vi "Set AQS.vi"(0 "NMR in":refnum<class "NMR.lvclass">, 5 "Number Samples":u16=5000 step=1, 7 "Units":u8(ring) items=["us", "ms"], 9 "Time Between Points":dbl min=0.0 step=1.0, 11 "error in (no error)":errorcluster) -> (4 "NMR out":refnum<class "NMR.lvclass">, 6 "Real Time":ext, 10 "String as ASCII":string, 15 "error out":errorcluster)   [LabVIEW 2011, in "NMR.lvclass"]
uses:
  NMR.lvclass
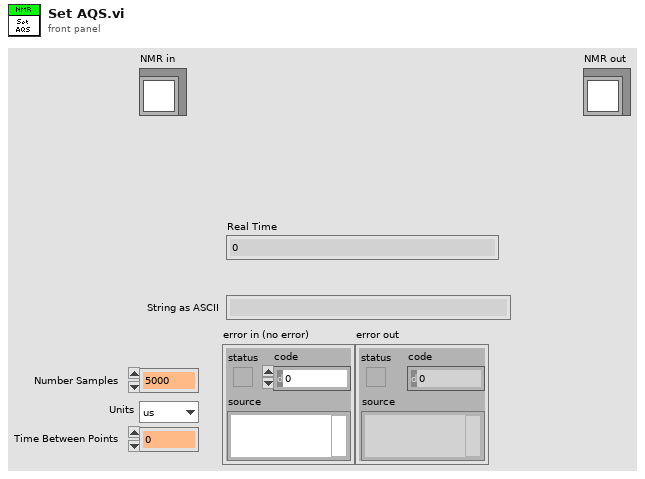
[diagram p1: front panel]
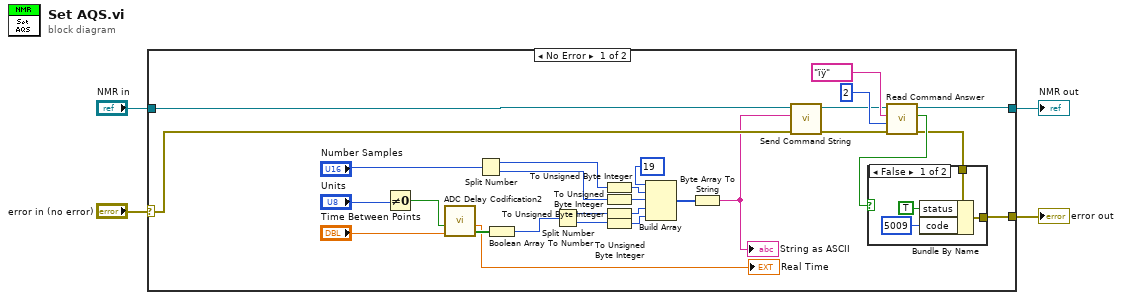
[diagram p0: block diagram]
diagram:
  n1 = case shown="No Error" "error in (no error)" {
    selector: "error in (no error)" -> [w31 w39]
    tunnel: [w5 w39] -> w3
    tunnel: [w7 w38] -> w1
    tunnel: "NMR in" -> [w32 w38]
    frame No Error {
      n2 = Not Equal To 0?(x="Units") -> (x != 0?=w9:bool)
      n3 = call "ADC Delay Codification2.vi"("Delay"="Time Between Points", "ms/us Delay"=w9) -> ("Final array"=w20:bool[], "Real Time"=→"Real Time":ext)  [unwired: 8 in]
      n4 = Split Number(x="Number Samples") -> (hi(x)=w14:u8, lo(x)=w13:u8)
      n5 = Boolean Array To Number(Boolean array=w20) -> (number=w17:u32)
      n6 = Split Number(x=w17) -> (hi(x)=w12:u16, lo(x)=w10:u16)
      n7 = To Unsigned Byte Integer(number=w14) -> (unsigned 8bit integer=w15:u8)
      n8 = To Unsigned Byte Integer(number=w13) -> (unsigned 8bit integer=w27:u8)
      n9 = To Unsigned Byte Integer(number=w12) -> (unsigned 8bit integer=w16:u8)
      n10 = To Unsigned Byte Integer(number=w10) -> (unsigned 8bit integer=w11:u8)
      n11 = Build Array(u32 19 ("element"), w15, w27, w16, w11) -> (w29:u32[])
      n12 = Byte Array To String(unsigned byte array=w29) -> (string=w26:string)
      "String as ASCII" <- w26
      n13 = call-dynamic "Send Command String.vi"("error in (no error)"=w31, "Command String"=w26, "NMR in"=w32) -> ("error out"=w30:errorcluster, "NMR out"=w6:refnum<class "NMR.lvclass">)  [unwired: 7 in]
      n14 = call-dynamic "Read Command Answer.vi"("error in (no error)"=w30, "bytes to read"=u32 2 ("Number bytes Read"), "String Seached"="ïÿ" ("search char"), "NMR in"=w6) -> ("error out"=w22:errorcluster, "Expected Answer?"=w23:bool, "NMR out"=w7:refnum<class "NMR.lvclass">)  [unwired: 5 in]
      n15 = case shown="False" w23 {
        tunnel: w22 -> [w34 w37]
        tunnel: [w33 w37] -> w5
        frame False {
          n16 = Bundle By Name(cluster=w34, "status"=TRUE, "code"=5009) -> (w33:errorcluster)
        }
        frame True {
        }
      }
    }
    frame Error {
    }
  }
  "error out" <- w3
  "NMR out" <- w1
